vi "Default VIP Aliases.vi"() -> (3 "Custom Aliases (empty = defaults only)":T1[](array[typedef])=[{"VIP String"="BSD 4-Clause", "SPDX IDs"=["BSD-4-Clause"]}, {"VIP String"="BSD", "SPDX IDs"=["BSD-3-Clause"]}, {"VIP String"="BSD License", "SPDX IDs"=["BSD-3-Clause"]}, {"VIP String"="BSD3", "SPDX IDs"=["BSD-3-Clause"]}, {"VIP String"="New BSD", "SPDX IDs"=["BSD-3-Clause"]}, {"VIP String"="BSD 2", "SPDX IDs"=["BSD-2-Clause"]}, {"VIP String"="BSD2", "SPDX IDs"=["BSD-2-Clause"]}, {"VIP String"="0-BSD", "SPDX IDs"=["0BSD"]}])   [LabVIEW 2017, in "VIP SBOM Support.lvlib"]
doc: "Provides a default mapping of VI Package License strings to SPDX license types based on commonly used license name formats in the VIPM package list."
uses:
  VIP SBOM Support.lvlib
  VIP License Alias.ctl
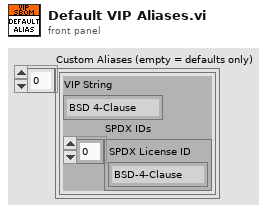
[diagram p1: front panel]
types:
  T1 = typedef "VIP SBOM Support.lvlib/VIP License Alias.ctl" = cluster{"VIP String":string, "SPDX IDs":string[]}
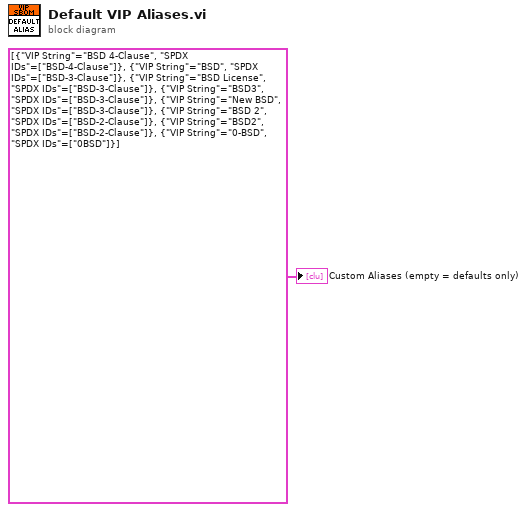
[diagram p0: block diagram]
diagram:
  "Custom Aliases (empty = defaults only)" <- T1[] [{"VIP String"="BSD 4-Clause", "SPDX IDs"=["BSD-4-Clause"]}, {"VIP String"="BSD", "SPDX IDs"=["BSD-3-Clause"]}, {"VIP String"="BSD License", "SPDX IDs"=["BSD-3-Clause"]}, {"VIP String"="BSD3", "SPDX IDs"=["BSD-3-Clause"]}, {"VIP String"="New BSD", "SPDX IDs"=["BSD-3-Clause"]}, {"VIP String"="BSD 2", "SPDX IDs"=["BSD-2-Clause"]}, {"VIP String"="BSD2", "SPDX IDs"=["BSD-2-Clause"]}, {"VIP String"="0-BSD", "SPDX IDs"=["0BSD"]}] ("Custom Aliases (empty = defaults only)")
